vi "hasServerCapability.vi"(8 "error in (no error)":errorcluster, 10 "Protocol ID in":string, 11 "IDeviceInfo in":refnum<class "IDeviceInfo.lvclass">) -> (0 "error out":errorcluster, 1 "hasCapability?":bool, 2 "Protocol ID out":string, 3 "IDeviceInfo out":refnum<class "IDeviceInfo.lvclass">)   [LabVIEW 2022 SP3, in "openDAQ.lvlib" / "IBaseObject.lvlib" / "IPropertyObject.lvlib" / "IDeviceInfo.lvlib" / "IDeviceInfo.lvclass"]
uses:
  <instrlib>/openDAQ/Public/Classes/IDeviceInfo/IDeviceInfo.lvclass
  <instrlib>/openDAQ/Public/Classes/IDeviceInfo/IDeviceInfo.lvclass/IDeviceInfo.ctl
  <instrlib>/openDAQ/Public/Classes/daqCoreTypes/IString/IString.lvclass
  <instrlib>/openDAQ/Binaries/Windows/x86/copendaq32.dll
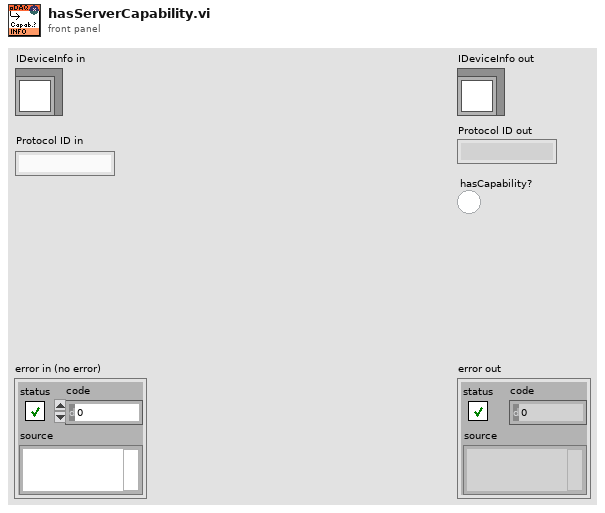
[diagram p1: front panel]
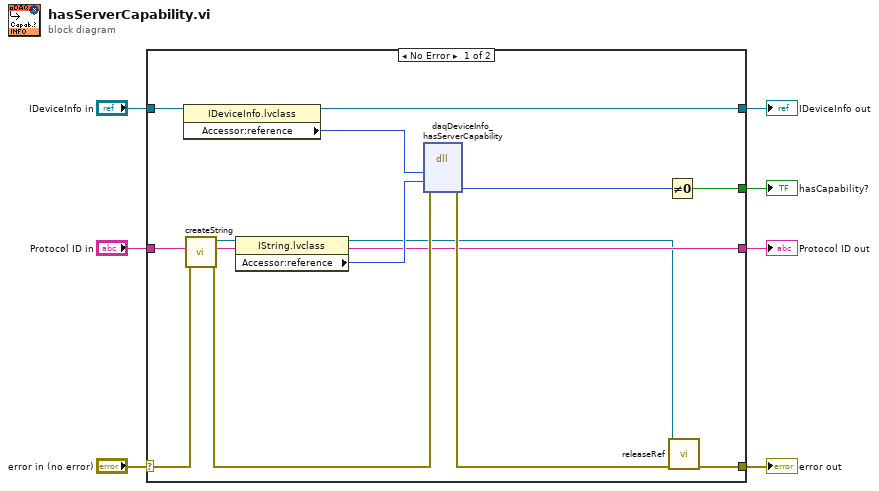
[diagram p0: block diagram]
diagram:
  n1 = case shown="No Error" "error in (no error)" {
    selector: "error in (no error)" -> [w11 w23]
    tunnel: [w9 w23] -> w6
    tunnel: [w14 w22] -> w4
    tunnel: "IDeviceInfo in" -> [w16 w22]
    tunnel: [w12 _] -> w3
    tunnel: "Protocol ID in" -> [w17 w21]
    tunnel: [w17 w21] -> w1
    frame No Error {
      n2 = property class="IDeviceInfo.lvclass"(reference=w16) -> (reference out=w14:refnum<class "IDeviceInfo.lvclass">, "Accessor:reference"=w15:i64)  [unwired: 1 in, 1 out]
      n3 = call <instrlib>:"createString.vi"("error in (no error)"=w11, "String"=w17) -> ("error out"=w19:errorcluster, "IString out"=w10:refnum<class "IString.lvclass">)  [unwired: 8 in]
      n4 = property class="IString.lvclass"(reference=w10) -> (reference out=w8:refnum<class "IString.lvclass">, "Accessor:reference"=w20:i64)  [unwired: 1 in, 1 out]
      n5 = dll-call lib="C:/Program Files (x86)/National Instruments/LabVIEW 2022/instr.lib/openDAQ/Binaries/Windows/x86/copendaq*.*" fn="daqDeviceInfo_hasServerCapability"(error in=w19, "deviceInfo"=w15, "protocolId"=w20) -> (error out=w18:errorcluster, "hasCapability"=w13:i64)  [unwired: 6 in, 1 out]
      n6 = Not Equal To 0?(x=w13) -> (x != 0?=w12:bool)
      n7 = call-dynamic "releaseRef.vi"("error in (no error)"=w18, "IBaseObject in"=w8) -> ("error out"=w9:errorcluster)  [unwired: 9 in]
    }
    frame Error {
    }
  }
  "error out" <- w6
  "IDeviceInfo out" <- w4
  "hasCapability?" <- w3
  "Protocol ID out" <- w1
